vi "utility.vi"() -> ()   [LabVIEW 2010]
uses:
  <vilib>/Analysis/polynomials.llb/Polynomial Plot (Samples).vi
  <vilib>/Analysis/NI_AALPro.lvlib
panel:
  in  "t offset (sec)":dbl=-0.89
  out "slope 4":dbl=0.000259124579638544
  out "slope 3":dbl=0.0008873535420112171
  out "slope 2":dbl=0.0010621643743997944
  out "intercept 4":dbl=0.000259124579638544
  out "intercept 3":dbl=0.0004568614899945912
  out "intercept 2":dbl=0.0007866636935624753
  out "intercept 1":dbl=0.001290866869319065
  out "slope":dbl=0.0017714964335866783
  out "1B-03-004 Measured Ramping vs. Measured Time":T1(graph)=[{"T ( sec )"=[2.006782435695, 3.002808172895, 3.994737620698, 5.009847295717, 5.995982965206, 7.032588859888, 8.002246666102, 8.993009580938999], "Ampliitudes 1"=[0.00470905, 0.00659808, 0.00843282, 0.0102004, 0.0121743, 0.0137404, 0.0152631, 0.0153594]}, {"T ( sec )"=[2.006782435695, 3.002808172895, 3.994737620698, 5.009847295717, 5.995982965206, 7.032588859888, 8.002246666102, 8.993009580938999], "Ampliitudes 1"=[0.00281843, 0.00393805, 0.00503484, 0.00616745, 0.00740345, 0.00835167, 0.0090163, 0.00916409]}, {"T ( sec )"=[2.006782435695, 3.002808172895, 3.994737620698, 5.009847295717, 5.995982965206, 7.032588859888, 8.002246666102, 8.993009580938999], "Ampliitudes 1"=[0.00226068, 0.0031143, 0.00398799, 0.00484602, 0.00585892, 0.00665268, 0.00757474, 0.00741362]}, {"T ( sec )"=[2.006782435695, 3.002808172895, 3.994737620698, 5.009847295717, 5.995982965206, 7.032588859888, 8.002246666102, 8.993009580938999], "Ampliitudes 1"=[0.000680395, 0.000917629, 0.00105338, 0.0013794, 0.00155139, 0.00176166, 0.00194577, 0.00195627]}, {"T ( sec )"=[0.0, 1.0, 2.0, 3.0, 4.0, 9.0], "Ampliitudes 1"=[0.001290866869319065, 0.0030623633029057433, 0.004833859736492422, 0.0066053561700791, 0.008376852603665778, 0.01723433477159917]}, {"T ( sec )"=[0.0, 1.0, 2.0, 3.0, 4.0, 9.0], "Ampliitudes 1"=[0.0007866636935624753, 0.0018488280679622698, 0.002910992442362064, 0.003973156816761859, 0.005035321191161653, 0.010346143063160625]}, {"T ( sec )"=[0.0, 1.0, 2.0, 3.0, 4.0, 9.0], "Ampliitudes 1"=[0.0004568614899945912, 0.0013442150320058083, 0.0022315685740170255, 0.0031189221160282422, 0.00400627565803946, 0.008443043368095544]}, {"T ( sec )"=[0.0, 1.0, 2.0, 3.0, 4.0, 9.0], "Ampliitudes 1"=[0.000259124579638544, 0.000472443261875277, 0.0006857619441120102, 0.0008990806263487432, 0.0011123993085854762, 0.0021789927197691417]}]
  in  "Ampliitudes 4":dbl[](array[numeric])=[0.000680395, 0.000917629, 0.00105338, 0.0013794, 0.00155139, 0.00176166, 0.00194577, 0.00195627]
  in  "Ampliitudes 3":dbl[](array[numeric])=[0.00226068, 0.0031143, 0.00398799, 0.00484602, 0.00585892, 0.00665268, 0.00757474, 0.00741362]
  in  "Ampliitudes 2":dbl[](array[numeric])=[0.00281843, 0.00393805, 0.00503484, 0.00616745, 0.00740345, 0.00835167, 0.0090163, 0.00916409]
  in  "Ampliitudes 1":dbl[](array[numeric])=[0.00470905, 0.00659808, 0.00843282, 0.0102004, 0.0121743, 0.0137404, 0.0152631, 0.0153594]
  in  "Measured T ( sec )":dbl[](array[numeric])=[2.896782435695, 3.892808172895, 4.884737620698, 5.899847295717, 6.885982965206, 7.922588859888, 8.892246666102, 9.883009580939]
  in  "Elapsed Time with offset ( sec ) 2":dbl
  in  "Elapsed Time with offset ( sec )":dbl
  in  "Ramp Duration msec":dbl
  in  "Full Amplitude 4 ( A )":dbl=2000.0
  in  "Full Amplitude 3 ( A )":dbl=5000.0
  in  "Current in":dbl=0.00667
  out "V out":dbl=5.0024999999999995
  out "1/R":dbl=0.0013333333333333333
  out "Current":dbl=0.006666666666666667
  in  "R":dbl=750.0
  in  "V":dbl=5.0
  out "Time 2-1 (Hz)":dbl=8112.968872810066
  out "Time 2-1 (sec)":dbl=0.00012325944
  in  "Time 2":dbl=0.000154
  in  "Time 1":dbl=3.074056e-05
  out "Sampling Frequency (Hz)":dbl=120000.0
  in  "Samples to Acquire":dbl=4000.0
  out "Total Pulse Wavefrom Period (ms)":dbl=0.03333333333333333
  out "Pulse Wavefrom Period (ms)":dbl=0.008333333333333333
  in  "Pulses":dbl=4.0
  in  "Pulse Wavefrom Freq (Hz)":dbl=120.0
  # "SET_PRGM_DEF > Program Frequency Index: 22 (i.e. 65Hz)"
  # "See 1B-03-004 \"Ramping\""
  # "-0.89"
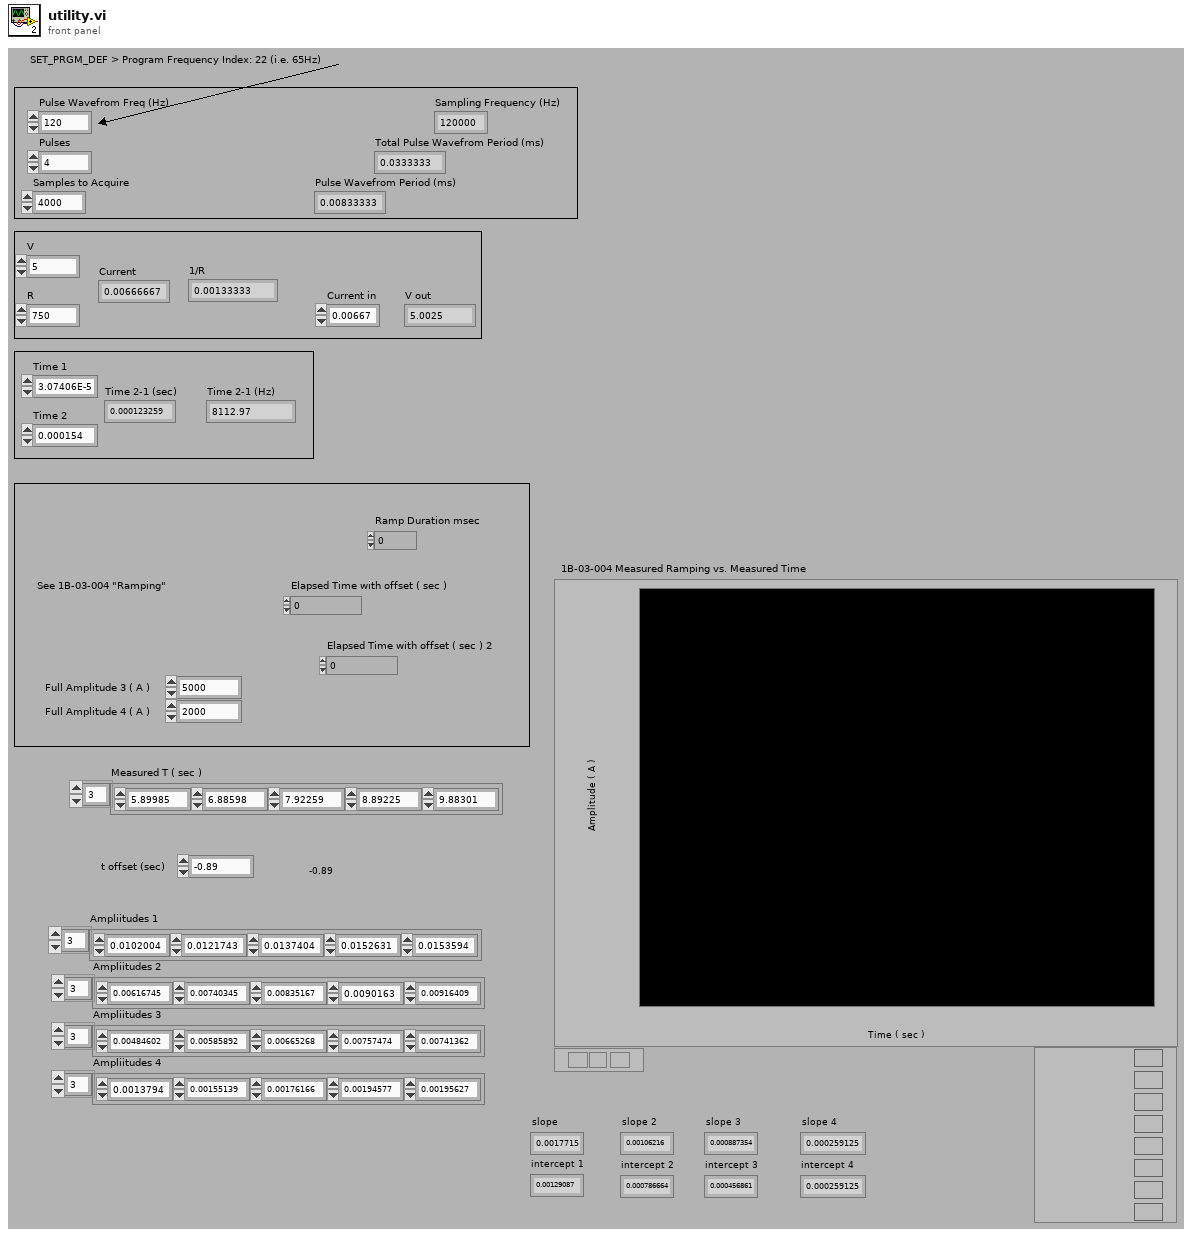
[diagram p1: front panel]
types:
  T1 = cluster{"T ( sec )":dbl[], "Ampliitudes 1":dbl[]}[]
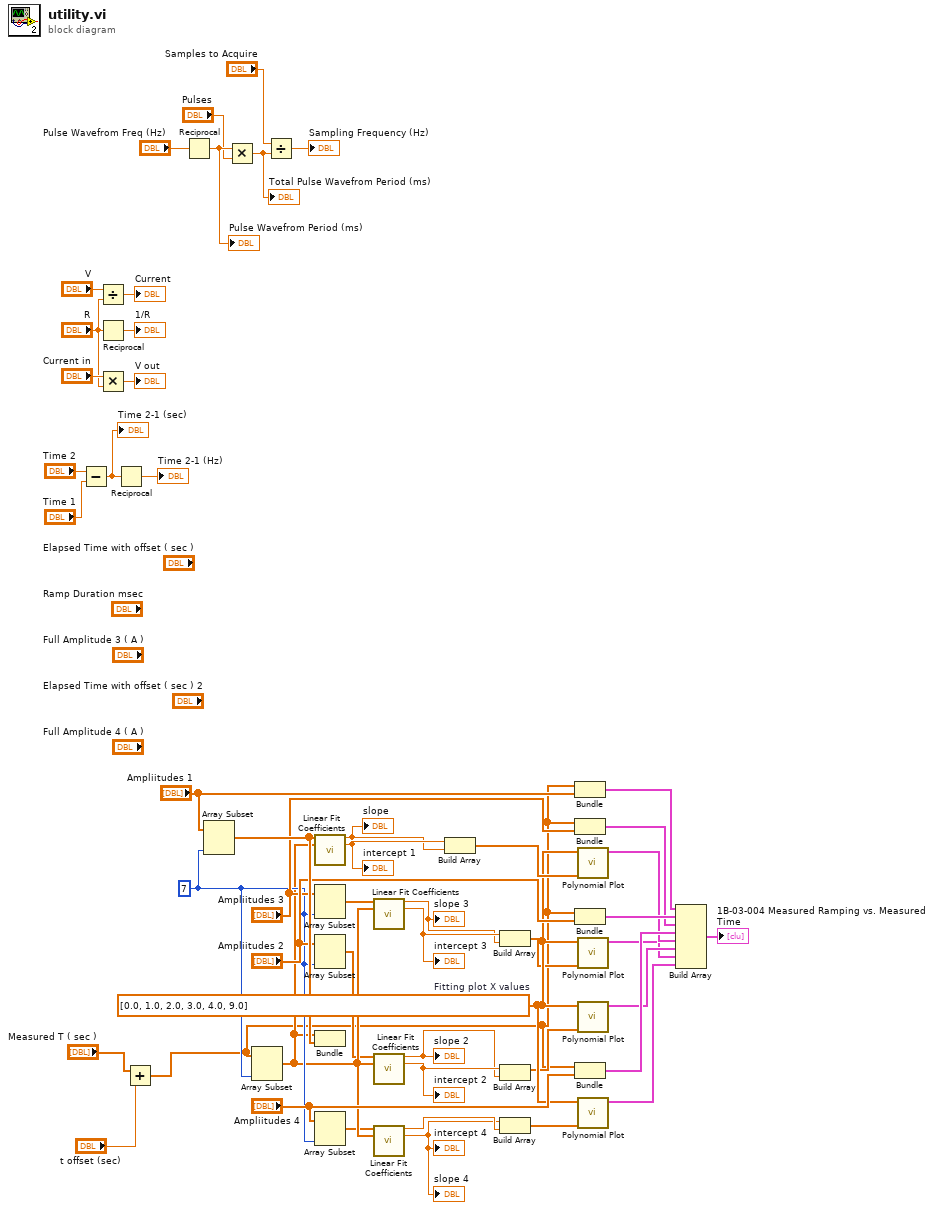
[diagram p0: block diagram]
diagram:
  w15 = dbl[] [0.0, 1.0, 2.0, 3.0, 4.0, 9.0]  # Fitting plot X values
  w21 = 7 ("length")
  n1 = Subtract(x="Time 2", y="Time 1") -> (x-y=w37:dbl)
  "Time 2-1 (sec)" <- w37
  n2 = Divide(x="V", y="R") -> (x/y=→"Current":dbl)
  n3 = Reciprocal(x="R") -> (1/x=→"1/R":dbl)
  n4 = Multiply(x="Current in", y="R") -> (x*y=→"V out":dbl)
  n5 = Reciprocal(x=w37) -> (1/x=→"Time 2-1 (Hz)":dbl)
  n6 = Add(x="Measured T ( sec )", y="t offset (sec)") -> (x+y=w1:dbl[])
  n7 = Reciprocal(x="Pulse Wavefrom Freq (Hz)") -> (1/x=w50:dbl)
  "Pulse Wavefrom Period (ms)" <- w50
  n8 = Array Subset(array="Ampliitudes 1", length=w21) -> (w29:dbl[])  [unwired: 1 in]
  n9 = Multiply(x=w50, y="Pulses") -> (x*y=w47:dbl)
  "Total Pulse Wavefrom Period (ms)" <- w47
  n10 = Array Subset(array=w1, length=w21) -> (w20:dbl[])  [unwired: 1 in]
  n11 = Divide(x="Samples to Acquire", y=w47) -> (x/y=→"Sampling Frequency (Hz)":dbl)
  n12 = call <vilib>:"Linear Fit Coefficients.vi"("Y"=w29, "X"=w20) -> ("slope"=w26:dbl, "intercept"=w27:dbl)  [unwired: 11 in, 1 out]
  "slope" <- w26
  "intercept 1" <- w27
  n13 = Array Subset(array="Ampliitudes 3", length=w21) -> (w18:dbl[])  [unwired: 1 in]
  n14 = Array Subset(array="Ampliitudes 2", length=w21) -> (w19:dbl[])  [unwired: 1 in]
  n15 = Bundle(w20, w29) -> ()  [unwired: 1 in, 1 out]
  n16 = Array Subset(array="Ampliitudes 4", length=w21) -> (w17:dbl[])  [unwired: 1 in]
  n17 = call <vilib>:"Linear Fit Coefficients.vi"("Y"=w18, "X"=w20) -> ("slope"=w4:dbl, "intercept"=w7:dbl)  [unwired: 11 in, 1 out]
  "intercept 3" <- w7
  "slope 3" <- w4
  n18 = call <vilib>:"Linear Fit Coefficients.vi"("Y"=w19, "X"=w20) -> ("slope"=w6:dbl, "intercept"=w8:dbl)  [unwired: 11 in, 1 out]
  "intercept 2" <- w8
  "slope 2" <- w6
  n19 = call <vilib>:"Linear Fit Coefficients.vi"("Y"=w17, "X"=w20) -> ("slope"=w16:dbl, "intercept"=w5:dbl)  [unwired: 11 in, 1 out]
  "intercept 4" <- w5
  "slope 4" <- w5
  n20 = Build Array(w27, w26) -> (w25:dbl[])
  n21 = Build Array(w7, w4) -> (w13:dbl[])
  n22 = Build Array(w8, w6) -> (w12:dbl[])
  n23 = Build Array(w5, w16) -> (w14:dbl[])
  n24 = Bundle(w1, "Ampliitudes 1"="Ampliitudes 1") -> (w35:cluster{dbl[], "Ampliitudes 1":dbl[]})  [unwired: 1 in]
  n25 = Bundle(w1, "Ampliitudes 3"="Ampliitudes 3") -> (w32:cluster{dbl[], "Ampliitudes 3":dbl[]})  [unwired: 1 in]
  n26 = Bundle(w1, "Ampliitudes 2"="Ampliitudes 2") -> (w33:cluster{dbl[], "Ampliitudes 2":dbl[]})  [unwired: 1 in]
  n27 = Bundle(w1, "Ampliitudes 4"="Ampliitudes 4") -> (w31:cluster{dbl[], "Ampliitudes 4":dbl[]})  [unwired: 1 in]
  n28 = call-poly <vilib>:"Polynomial Plot.vi"("P(x)"=w25, "X"=w15) -> ("polynomial plot"=w28:cluster{dbl[], "P(A)":dbl[]})  [unwired: 8 in, 1 out]
  n29 = call-poly <vilib>:"Polynomial Plot.vi"("P(x)"=w13, "X"=w15) -> ("polynomial plot"=w10:cluster{dbl[], "P(A)":dbl[]})  [unwired: 8 in, 1 out]
  n30 = call-poly <vilib>:"Polynomial Plot.vi"("P(x)"=w12, "X"=w15) -> ("polynomial plot"=w11:cluster{dbl[], "P(A)":dbl[]})  [unwired: 8 in, 1 out]
  n31 = call-poly <vilib>:"Polynomial Plot.vi"("P(x)"=w14, "X"=w15) -> ("polynomial plot"=w9:cluster{dbl[], "P(A)":dbl[]})  [unwired: 8 in, 1 out]
  n32 = Build Array(w35, w33, w32, w31, w28, w11, w10, w9) -> (→"1B-03-004 Measured Ramping vs. Measured Time":cluster{dbl[], "P(A)":dbl[]}[])
